vi "PE7265_Manage_Monitor.vi"(3 "Lockin# (in)":u16, 4 "System Monitor Variables (in)":T1, 5 "Global-Status (in)":T2={"Lockin 1"=[], "X1-Display"=0.0, "X1 Percent"=0.0, "Y1-Display"=0.0, "X1 Percent 2"=0.0, "Unit X1"="nV", "Unit X1a"="nV", "Unit X2"="nV", "Unit X2a"="nV", "X1 Overload"=FALSE, "Y1 Overload"=FALSE, "Sensitivity Setpoint"=26, "X1"=0.0, "Y1"=0.0} {"Sensitivity Setpoint" items=["2 nV", "5 nV", "10 nV", "20 nV", "50 nV", "100 nV", "200 nV", "500 nV", "1 µV", "2 µV", "5 µV", "10 µV", "20 µV", "50 µV", "100 µV", "200 µV", "500 µV", "1 mV", "2 mV", "5 mV", "10 mV", "20 mV", "50 mV", "100 mV", "200 mV", "500 mV", "1 V", ""]; "X1 Percent 2" scale=0.0..1.0; "X1 Percent" scale=0.0..1.0; "X1-Display" format="%#4_5f"}, 6 "Command (in)":T2={"Lockin 1"=[], "X1-Display"=0.0, "X1 Percent"=0.0, "Y1-Display"=0.0, "X1 Percent 2"=0.0, "Unit X1"="nV", "Unit X1a"="nV", "Unit X2"="nV", "Unit X2a"="nV", "X1 Overload"=FALSE, "Y1 Overload"=FALSE, "Sensitivity Setpoint"=26, "X1"=0.0, "Y1"=0.0} {"Sensitivity Setpoint" items=["2 nV", "5 nV", "10 nV", "20 nV", "50 nV", "100 nV", "200 nV", "500 nV", "1 µV", "2 µV", "5 µV", "10 µV", "20 µV", "50 µV", "100 µV", "200 µV", "500 µV", "1 mV", "2 mV", "5 mV", "10 mV", "20 mV", "50 mV", "100 mV", "200 mV", "500 mV", "1 V", ""]; "X1 Percent 2" scale=0.0..1.0; "X1 Percent" scale=0.0..1.0; "X1-Display" format="%#4_5f"}, 7 "queue (in)":refnum<queue>) -> (0 "System Monitor Variables (out)":T1, 1 "Monitor (out)":T2={"Lockin 1"=[], "X1-Display"=0.0, "X1 Percent"=0.0, "Y1-Display"=0.0, "X1 Percent 2"=0.0, "Unit X1"="nV", "Unit X1a"="nV", "Unit X2"="nV", "Unit X2a"="nV", "X1 Overload"=FALSE, "Y1 Overload"=FALSE, "Sensitivity Setpoint"=26, "X1"=0.0, "Y1"=0.0} {"Sensitivity Setpoint" items=["2 nV", "5 nV", "10 nV", "20 nV", "50 nV", "100 nV", "200 nV", "500 nV", "1 µV", "2 µV", "5 µV", "10 µV", "20 µV", "50 µV", "100 µV", "200 µV", "500 µV", "1 mV", "2 mV", "5 mV", "10 mV", "20 mV", "50 mV", "100 mV", "200 mV", "500 mV", "1 V", ""]; "X1 Percent 2" scale=0.0..1.0; "X1 Percent" scale=0.0..1.0; "X1-Display" format="%#4_5f"})   [LabVIEW 2019]
uses:
  PE7265/PE7265-Cluster.ctl
  Global/Global Variables/System Monitor Cluster.ctl
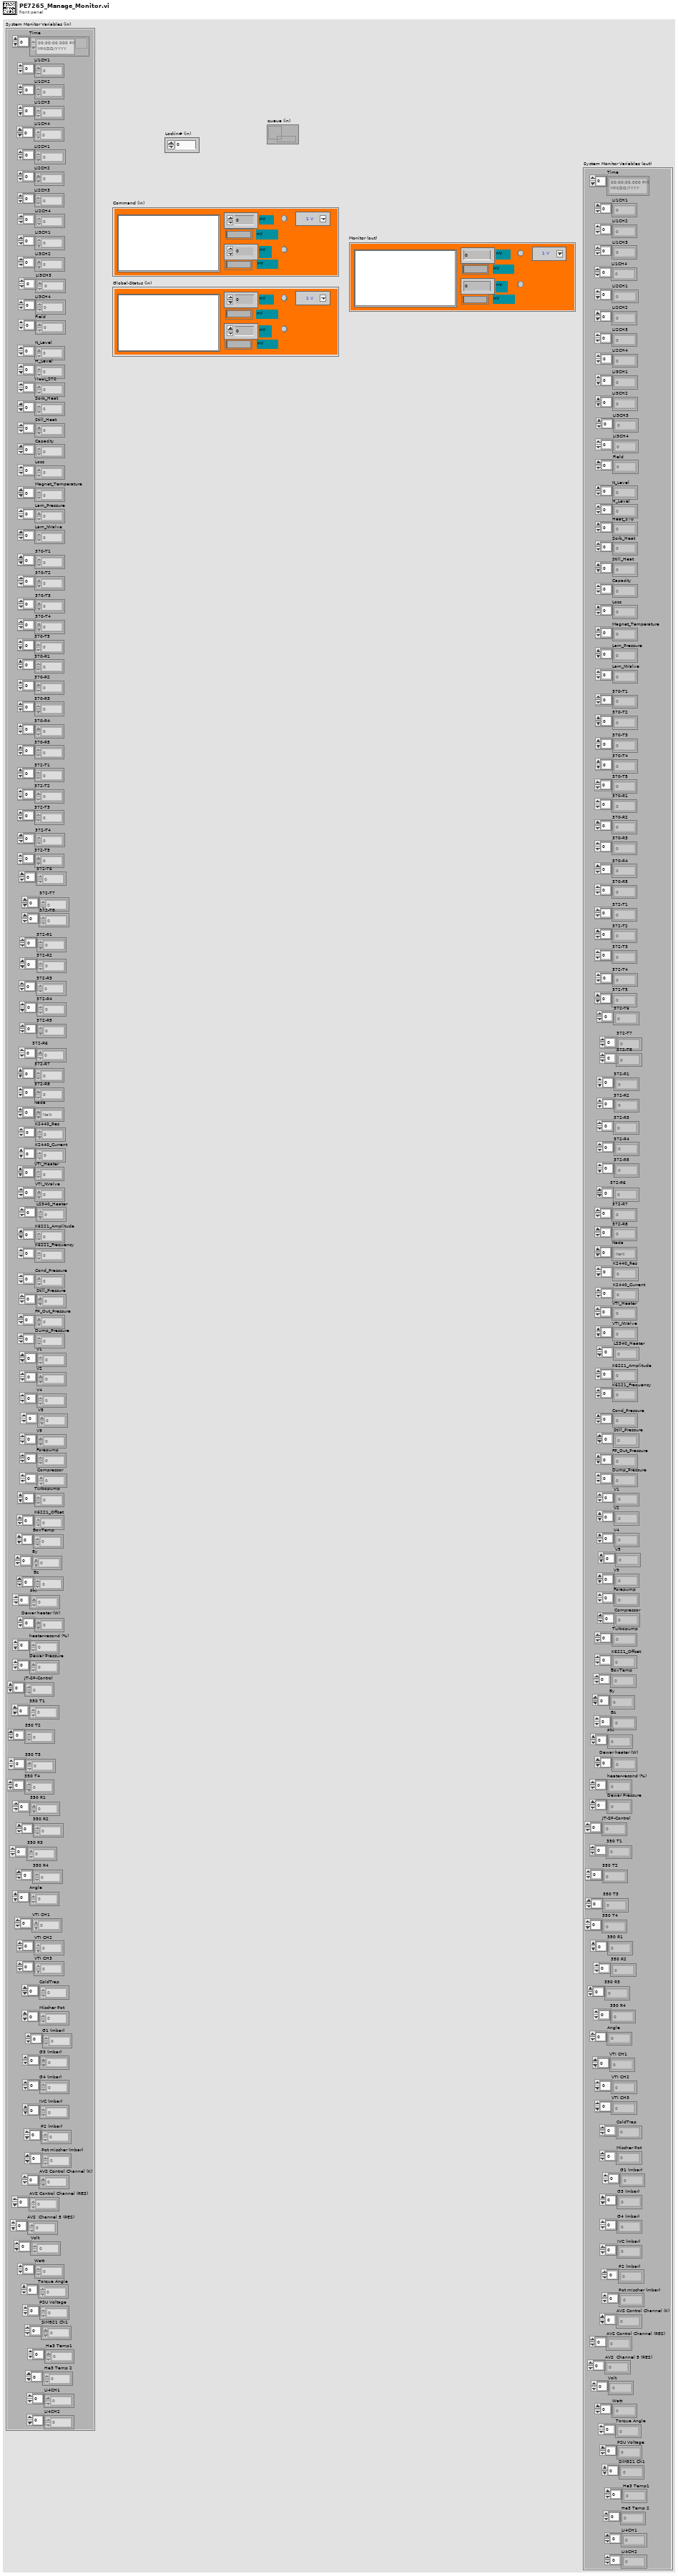
[diagram p1: front panel]
types:
  T1 = typedef "System Monitor Cluster.ctl" = cluster{"Time":timestamp[], "LI1CH1":dbl[], "LI1CH2":dbl[], "LI2CH1":dbl[], "LI2CH2":dbl[], "LI3CH1":dbl[], "LI3CH2":dbl[], "Field":dbl[], "N_Level":dbl[], "H_Level":dbl[], "Heat_370":dbl[], "Sorb_Heat":dbl[], "Still_Heat":dbl[], "Capacity":dbl[], "Loss":dbl[], "Magnet_Temperature":dbl[], "Lam_Pressure":dbl[], "Lam_NValve":dbl[], "370-T1":dbl[], "370-T2":dbl[], "370-T3":dbl[], "370-T4":dbl[], "370-T5":dbl[], "370-R1":dbl[], "370-R2":dbl[], "370-R3":dbl[], "370-R4":dbl[], "370-R5":dbl[], "372-T1":dbl[], "372-T2":dbl[], "372-T3":dbl[], "372-T4":dbl[], "372-T5":dbl[], "372-T6":dbl[], "372-R1":dbl[], "372-R2":dbl[], "372-R3":dbl[], "372-R4":dbl[], "372-R5":dbl[], "372-R6":dbl[], "Nada":dbl[], "K2440_Res":dbl[], "K2440_Current":dbl[], "VTI_Heater":dbl[], "VTI_NValve":dbl[], "LS340_Heater":dbl[], "K6221_Amplitude":dbl[], "K6221_Frequency":dbl[], "Cond_Pressure":dbl[], "Still_Pressure":dbl[], "FP_Out_Pressure":dbl[], "Dump_Pressure":dbl[], "V1":dbl[], "V2":dbl[], "V4":dbl[], "V5":dbl[], "V9":dbl[], "Forepump":dbl[], "Compressor":dbl[], "K6221_Offset":dbl[], "BoxTemp":dbl[], "By":dbl[], "Bz":dbl[], "Phi":dbl[], "heater-recond (%)":dbl[], "Dewar Pressure ":dbl[], "JT-SP-Control":dbl[], "350 T1":dbl[], "350 T2":dbl[], "350 T3":dbl[], "350 T4":dbl[], "350 R1":dbl[], "350 R2":dbl[], "350 R3":dbl[], "350 R4":dbl[], "Angle":dbl[], "VTI CH1":dbl[], "VTI CH2":dbl[], "VTI CH3":dbl[], "ColdTrap":dbl[], "Mischer Pot":dbl[], "G1 (mbar)":dbl[], "G3 (mbar) ":dbl[], "G4 (mbar)":dbl[], "IVC (mbar)":dbl[], "P2 (mbar) ":dbl[], "Pot mischer (mbar)":dbl[], "AVS Control Channel (K)":dbl[], "AVS Control Channel (RES)":dbl[], "AVS  Channel 5 (RES) ":dbl[], "LI3CH3":dbl[], "LI3CH4":dbl[], "LI1CH3":dbl[], "LI1CH4":dbl[], "LI2CH3":dbl[], "LI2CH4":dbl[], "Volt":dbl[], "Watt":dbl[], "Torque Angle":dbl[], "Dewar heater (W)":dbl[], "PSU Voltage":dbl[], "Turbopump":dbl[], "372-R7":dbl[], "372-T7":dbl[], "SIM921 Ch1":dbl[], " He3 Temp1":dbl[], " He3 Temp 2":dbl[], "LI4CH1":dbl[], "LI4CH2":dbl[], "372-T8":dbl[], "372-R8":dbl[]}
  T2 = typedef "PE7265-Cluster.ctl" = cluster{"Lockin 1":dbl[][], "X1-Display":dbl, "X1 Percent":dbl, "Y1-Display":dbl, "X1 Percent 2":dbl, "Unit X1":string, "Unit X1a":string, "Unit X2":string, "Unit X2a":string, "X1 Overload":bool, "Y1 Overload":bool, "Sensitivity Setpoint":i16, "X1":dbl, "Y1":dbl}
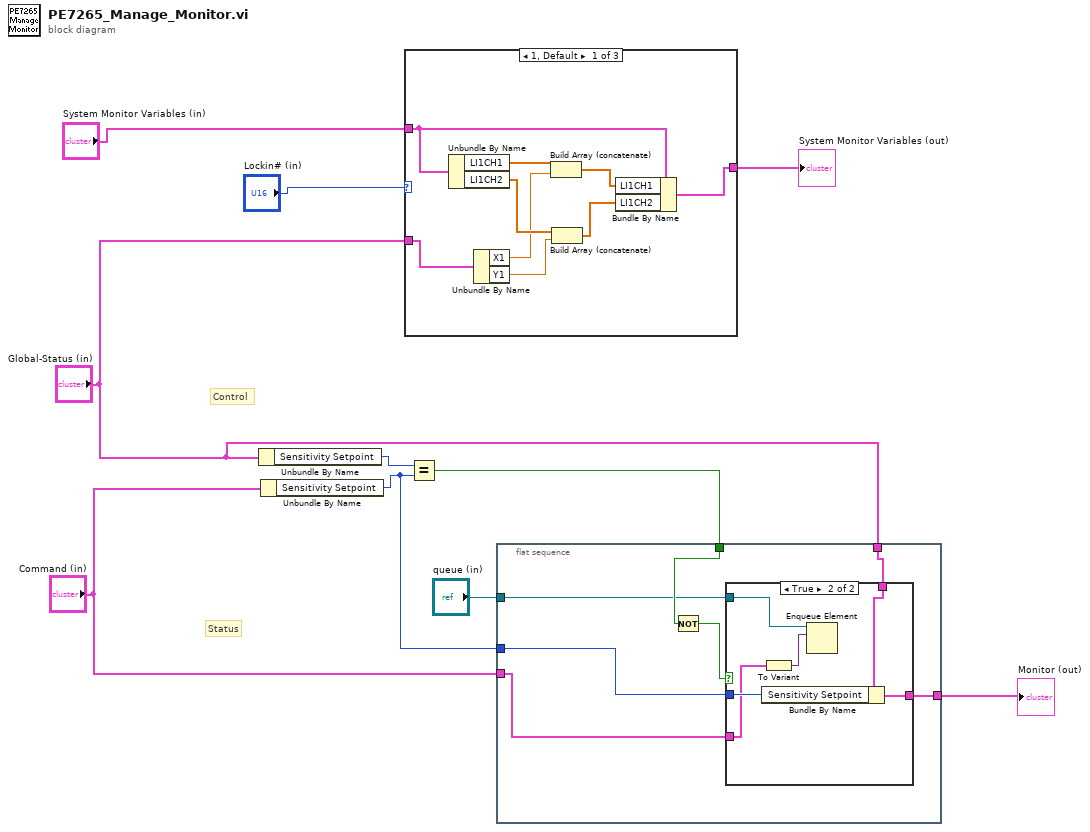
[diagram p0: block diagram]
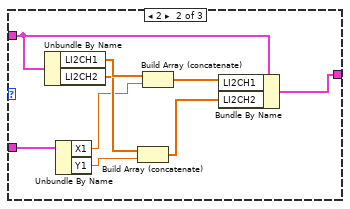
[diagram p3: hidden frame]
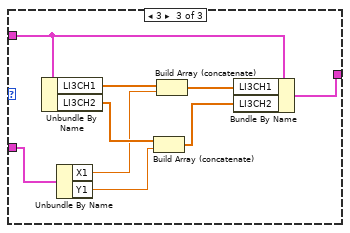
[diagram p4: hidden frame]
diagram:
  # "Status"
  # "Control"
  n1 = Unbundle By Name("Global-Status (in)") -> ("Sensitivity Setpoint"=w7:i16)
  n2 = Unbundle By Name("Command (in)") -> ("Sensitivity Setpoint"=w5:i16)
  n3 = case shown="1, Default" "Lockin# (in)" {
    tunnel: "System Monitor Variables (in)" -> [w18 w28 w36]
    tunnel: [w17 w26 w37] -> w8
    tunnel: "Global-Status (in)" -> [w19 w27 w33]
    frame 1, Default {
      n4 = Unbundle By Name(w18) -> ("LI1CH1"=w16:dbl[], "LI1CH2"=w15:dbl[])
      n5 = Unbundle By Name(w19) -> ("X1"=w14:dbl, "Y1"=w13:dbl)
      n6 = Build Array (concatenate)(w16, w14) -> (w12:dbl[])
      n7 = Build Array (concatenate)(w15, w13) -> (w11:dbl[])
      n8 = Bundle By Name(cluster=w18, "LI1CH1"=w12, "LI1CH2"=w11) -> (w17:T1)
    }
    frame 2 {
      n9 = Unbundle By Name(w28) -> ("LI2CH1"=w25:dbl[], "LI2CH2"=w24:dbl[])
      n10 = Unbundle By Name(w27) -> ("X1"=w23:dbl, "Y1"=w22:dbl)
      n11 = Build Array (concatenate)(w24, w22) -> (w20:dbl[])
      n12 = Build Array (concatenate)(w25, w23) -> (w21:dbl[])
      n13 = Bundle By Name(cluster=w28, "LI2CH1"=w21, "LI2CH2"=w20) -> (w26:T1)
    }
    frame 3 {
      n14 = Unbundle By Name(w36) -> ("LI3CH1"=w35:dbl[], "LI3CH2"=w34:dbl[])
      n15 = Unbundle By Name(w33) -> ("X1"=w32:dbl, "Y1"=w31:dbl)
      n16 = Build Array (concatenate)(w34, w31) -> (w29:dbl[])
      n17 = Build Array (concatenate)(w35, w32) -> (w30:dbl[])
      n18 = Bundle By Name(cluster=w36, "LI3CH1"=w30, "LI3CH2"=w29) -> (w37:T1)
    }
  }
  "System Monitor Variables (out)" <- w8
  n19 = Equal?(x=w7, y=w5) -> (x = y?=w4:bool)
  n20 = flat-sequence {
    tunnel: "Command (in)" -> [w39]
    tunnel: w5 -> [w42]
    tunnel: w4 -> [w41]
    tunnel: "Global-Status (in)" -> [w44]
    tunnel: [w43] -> w2
    tunnel: "queue (in)" -> [w38]
    frame #0 {
      n21 = Not(x=w41) -> (.not. x?=w40:bool)
      n22 = case shown="True" w40 {
        tunnel: w44 -> [w45 w51]
        tunnel: [w45 w50] -> w43
        tunnel: w42 -> [_ w49]
        tunnel: w39 -> [_ w48]
        tunnel: w38 -> [_ w46]
        frame False {
        }
        frame True {
          n23 = Bundle By Name(cluster=w51, "Sensitivity Setpoint"=w49) -> (w50:T2)
          n24 = To Variant(anything=w48) -> (Variant=w47:variant)
          n25 = Enqueue Element(queue=w46, element=w47) -> ()  [unwired: 2 in, 3 out]
        }
      }
    }
  }
  "Monitor (out)" <- w2
